vi "delStartup.vi"(0 "object in":refnum<class "interface.lvclass">, 1 "启动文件路径":path, 5 "error in (no error)":errorcluster) -> (14 "object out":refnum<class "interface.lvclass">, 15 "删除标记":bool, 19 "error out":errorcluster)   [LabVIEW 2016, in "interface.lvclass"]
uses:
  interface.lvclass
  <vilib>/registry/registry.llb/Registry RtKey.ctl
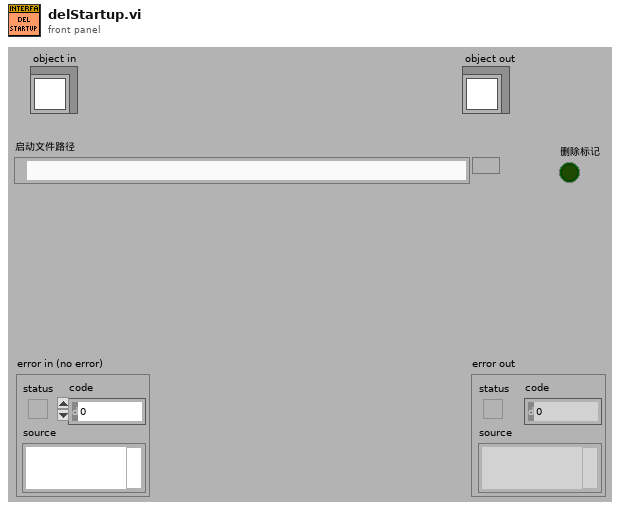
[diagram p1: front panel]
types:
  T1 = typedef "Registry RtKey.ctl" = enum32{"HKEY_CLASSES_ROOT", "HKEY_CURRENT_USER", "HKEY_LOCAL_MACHINE", "HKEY_USERS", "HKEY_PERFORMANCE_DATA", "HKEY_CURRENT_CONFIG", "HKEY_DYN_DATA"}
  T2 = typedef "Registry refnum.ctl" = refnum<k1>
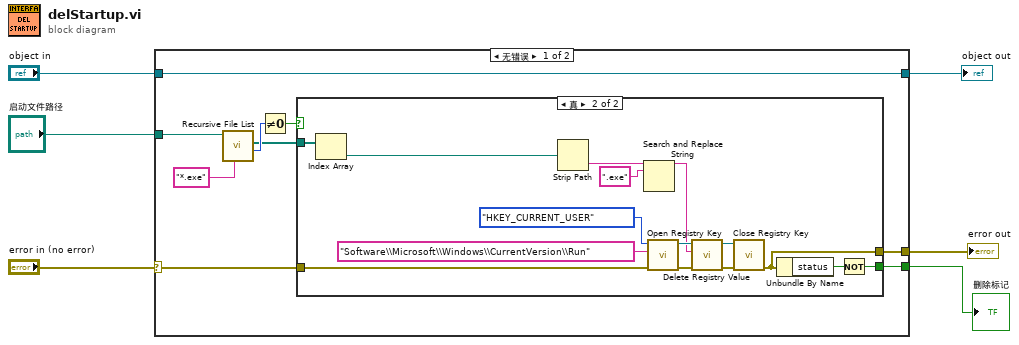
[diagram p0: block diagram]
diagram:
  n1 = case shown="无错误" "error in (no error)" {
    selector: "error in (no error)" -> [w8 w33]
    tunnel: [w9 w33] -> w5
    tunnel: [w15 w32] -> w3
    tunnel: "object in" -> [w15 w32]
    tunnel: [w10 _] -> w2
    tunnel: "启动文件路径" -> [w7 _]
    frame No Error {
      n2 = call <vilib>:"Recursive File List.vi"("pattern"="*.exe", "Folder Path"=w7) -> ("Number of Files"=w13:i32, "All Files in Dir"=w12:path[])  [unwired: 5 in, 3 out]
      n3 = Not Equal To 0?(x=w13) -> (x != 0?=w14:bool)
      n4 = case shown="真" w14 {
        tunnel: w12 -> [_ w31]
        tunnel: [_ w20] -> w10
        tunnel: [w16 w18] -> w9
        tunnel: w8 -> [w16 w17]
        frame False {
        }
        frame True {
          n5 = Index Array(array=w31) -> (element=w30:path)  [unwired: 1 in]
          n6 = Strip Path(path=w30) -> (name=w29:string)  [unwired: 1 out]
          n7 = Search and Replace String(input string=w29, search string=".exe" ("搜索字符串")) -> (result string=w19:string)  [unwired: 6 in, 3 out]
          n8 = call <vilib>:"Open Registry Key.vi"("error in (no error)"=w17, "subkey"="Software\\Microsoft\\Windows\\CurrentVersion\\Run", "root key (HKEY_LOCAL_MACHINE)"=Registry_RtKey."HKEY_CURRENT_USER") -> ("error out"=w23:errorcluster, "refnum out"=w25:T2)  [unwired: 7 in]
          n9 = call <vilib>:"Delete Registry Value.vi"("error in (no error)"=w23, "value"=w19, "refnum"=w25) -> ("error out"=w22:errorcluster, "refnum out"=w24:T2)  [unwired: 7 in]
          n10 = call <vilib>:"Close Registry Key.vi"("error in (no error)"=w22, "refnum"=w24) -> ("error out"=w18:errorcluster)  [unwired: 5 in]
          n11 = Unbundle By Name(w18) -> ("status"=w21:bool)
          n12 = Not(x=w21) -> (.not. x?=w20:bool)
        }
      }
    }
    frame Error {
    }
  }
  "error out" <- w5
  "object out" <- w3
  "删除标记" <- w2
